vi "GSM_SPUR_RESULT.vi"(0 "Session In":refnum<visa-resource-name>="TCPIP0::K-N90X0A-00005.local::inst0::INSTR", 11 "error in":errorcluster {"code" format="%.0x"}) -> (4 "Session Out":refnum<visa-resource-name>, 8 "array w/ subset deleted":dbl[](array[numeric]), 15 "error out":errorcluster {"code" format="%.0x"})   [LabVIEW 2018]
doc: "Launches the Instrument I/O Assistant, which you can use to communicate with message-based instruments and graphically parse the response. For example you can communicate with an instrument that uses a serial, Ethernet, or GPIB interface."
panel:
  out "spreadsheet string":string
  in  "Timeout":u32=3000
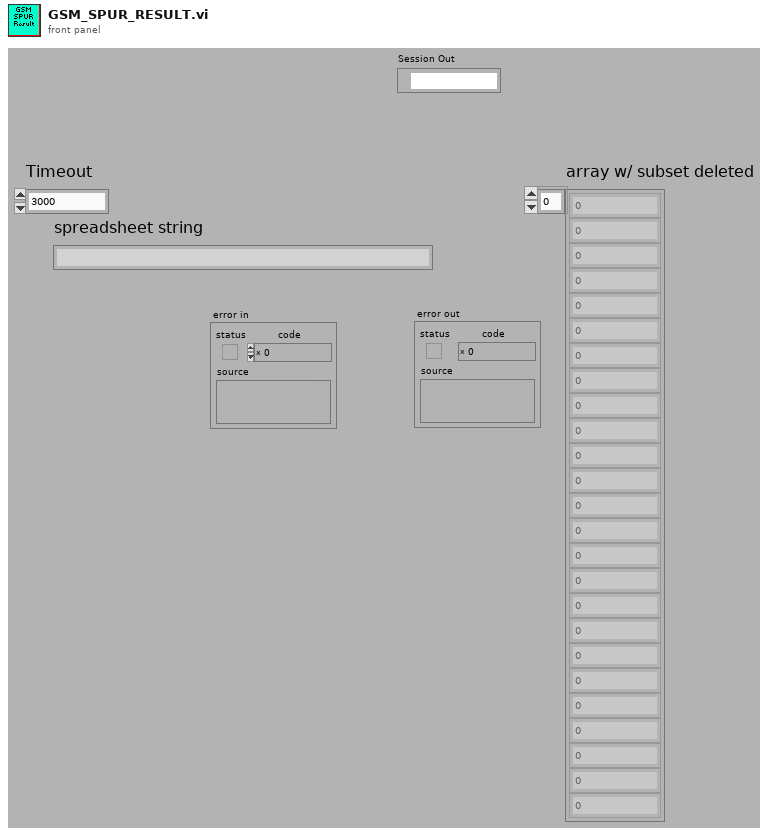
[diagram p1: front panel]
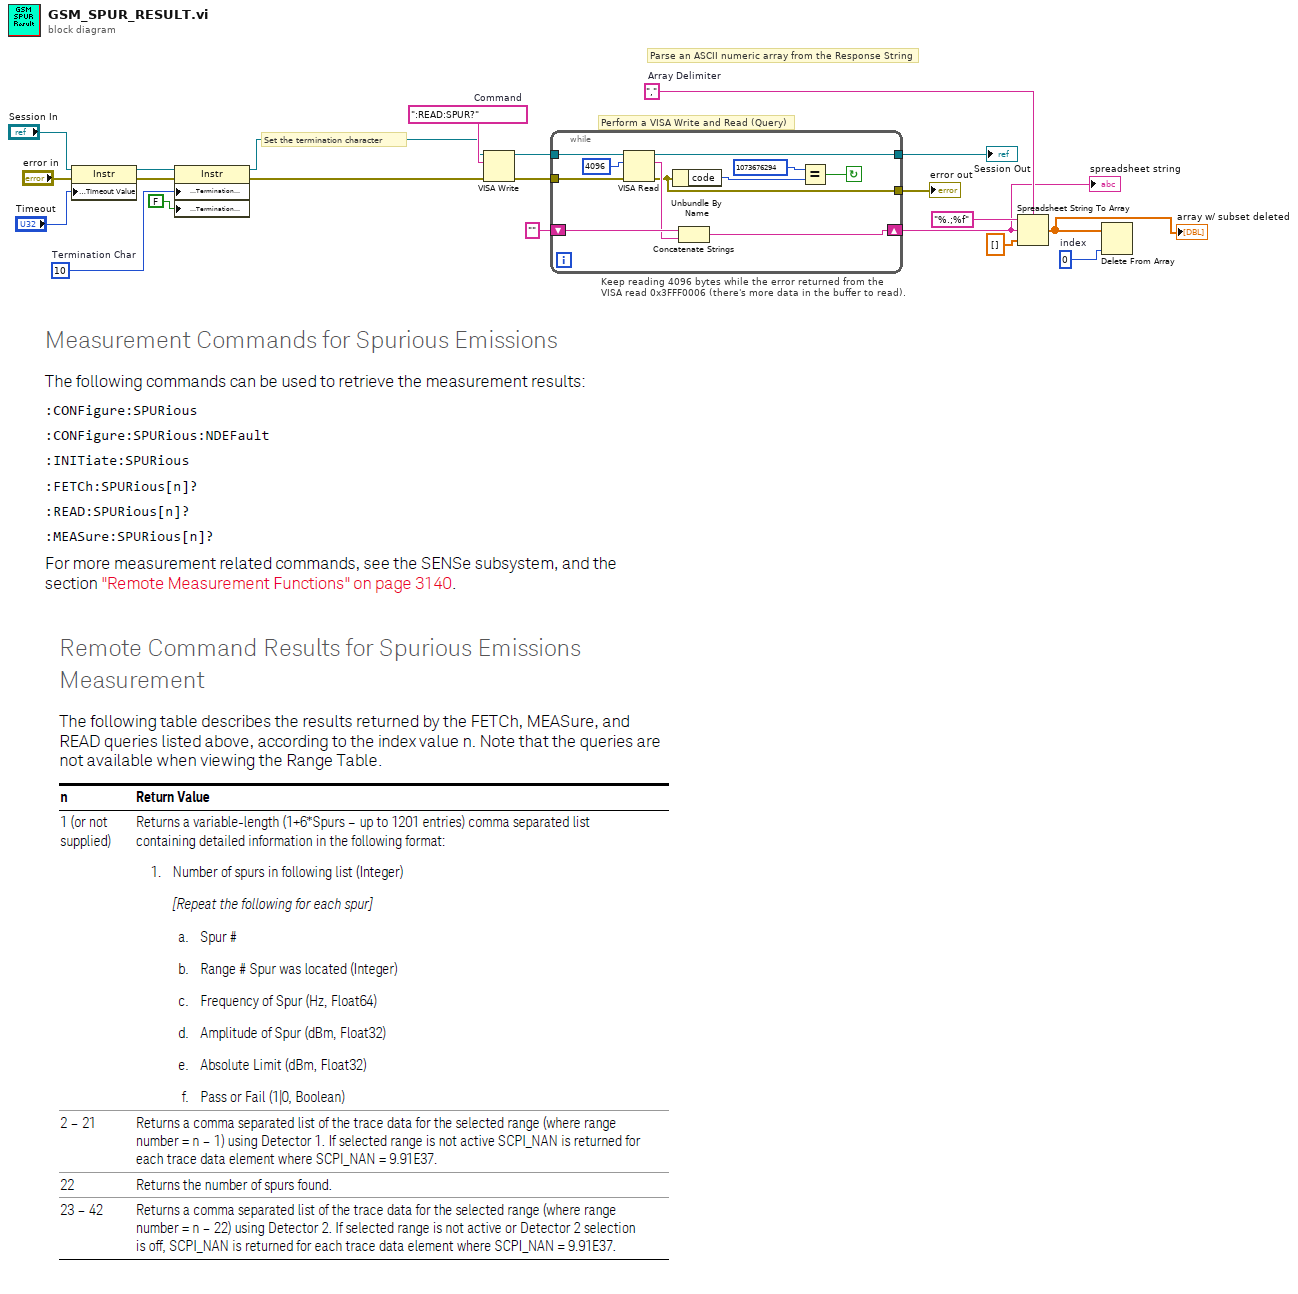
[diagram p0: block diagram]
diagram:
  w11 = ":READ:SPUR?"  # Command
  w5 = 0  # index
  w8 = ","  # Array Delimiter
  w18 = u8 10  # Termination Char
  # "Parse an ASCII numeric array from the Response String"
  # "Perform a VISA Write and Read (Query)"
  # "Keep reading 4096 bytes while the error returned from the\nVISA read 0x3FFF0006 (there's more data in the buffer to read)."
  # "Set the termination character"
  n1 = property class="Instr"(reference="Session In", error in="error in", "General Settings:Timeout Value"="Timeout") -> (reference out=w17:refnum<visa-resource-name>, error out=w19:errorcluster)
  n2 = property class="Instr"(reference=w17, error in=w19, "Message Based Settings:Termination Character"=w18, "Message Based Settings:Termination Character Enable"=FALSE ("enable")) -> (reference out=w3:refnum<visa-resource-name>, error out=w4:errorcluster)
  n3 = VISA Write(VISA resource name=w3, write buffer=w11, error in (no error)=w4) -> (VISA resource name out=w15:refnum<visa-resource-name>, error out=w14:errorcluster)  [unwired: 1 out]
  n4 = while {
    tunnel: w15 -> [w29]
    shift-right: [w23] -> w2
    shift-left: "" -> [w28]
    tunnel: w14 -> [w26]
    tunnel: [w25] -> w13
    tunnel: [w22] -> w7
    stop <- w24 continue-if-true
    n5 = VISA Read(VISA resource name=w29, byte count=u32 4096 ("byte count (0)"), error in (no error)=w26) -> (VISA resource name out=w22:refnum<visa-resource-name>, read buffer=w27:string, error out=w25:errorcluster)  [unwired: 1 out]
    n6 = Unbundle By Name(w25) -> ("code"=w31:i32)
    n7 = Concatenate Strings(w28, w27) -> (w23:string)
    n8 = Equal?(x=1073676294, y=w31) -> (x = y?=w24:bool)
  }
  "error out" <- w13
  "Session Out" <- w7
  "spreadsheet string" <- w2
  n9 = Spreadsheet String To Array(delimiter (Tab)=w8, format string="%.;%f", spreadsheet string=w2, array type (2D Dbl)=dbl[] []) -> (array=w1:dbl[])
  "array w/ subset deleted" <- w1
  n10 = Delete From Array(array=w1, index=w5) -> ()  [unwired: 1 in, 2 out]
